vi "读写键段.vi"(7 "枚举":enum16{"write", "read", "读键", "读段"}(ring), 8 "值":string, 9 "key":string caption="键", 10 "段":string, 11 "配置文件":path=path "D:/Labviewprogram/多账户登录") -> (0 "读取值":string, 1 "键名":string[](array[string]) caption="获取键名", 2 "获取段名":string[](array[string]))   [LabVIEW 2018]
uses:
  <vilib>/Utility/config.llb/Write Key (String).vi
  <vilib>/Utility/config.llb/Read Key (String).vi
  <vilib>/Utility/config.llb/NI_LVConfig.lvlib
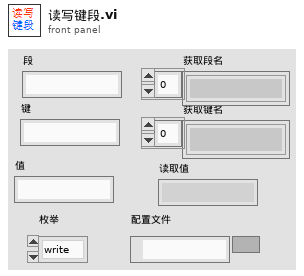
[diagram p1: front panel]
types:
  T1 = typedef "NI_LVConfig.lvlib/Config Data RefNum.ctl" = refnum<k1>
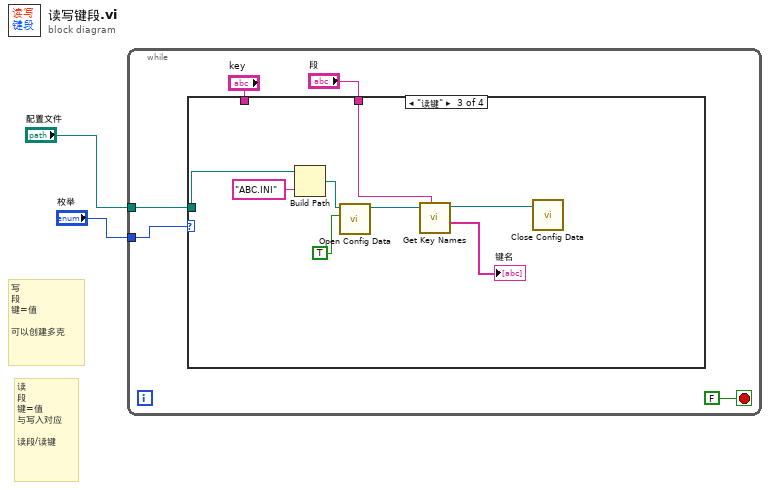
[diagram p0: block diagram]
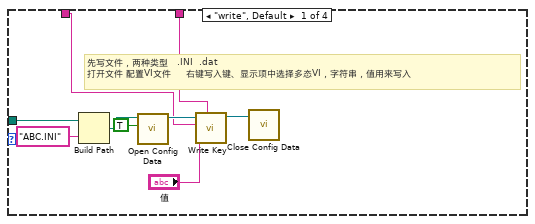
[diagram p2: hidden frame]
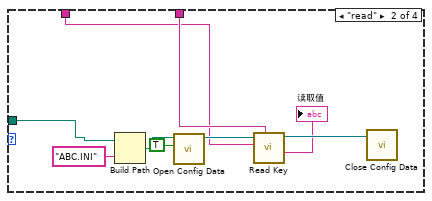
[diagram p3: hidden frame]
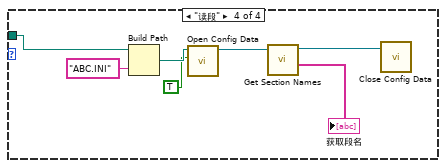
[diagram p4: hidden frame]
diagram:
  # "读\n段\n键=值\n与写入对应\n\n读段/读键"
  # "写\n段\n键=值\n\n可以创建多克"
  n1 = while {
    tunnel: "配置文件" -> [w5]
    tunnel: "枚举" -> [w6]
    stop <- FALSE stop-if-true
    n2 = case shown="\"读键\"" w6 {
      tunnel: w5 -> [w16 w20 w32 w34]
      tunnel: "段" -> [w10 w19 w27 _]
      tunnel: "key" -> [w9 w18 _ _]
      frame "write", Default {
        # "先写文件，两种类型   .INI  .dat\n打开文件 配置VI文件     右键写入键、显示项中选择多态VI，字符串，值用来写入"
        n3 = Build Path(base path=w16, name or relative path="ABC.INI" ("名称或相对路径")) -> (appended path=w14:path)
        n4 = call <vilib>:"Open Config Data.vi"("create file if necessary (T)"=TRUE, "configuration file path"=w14) -> ("refnum"=w13:T1)  [unwired: 7 in, 2 out]
        n5 = call-poly <vilib>:"Write Key.vi"("section"=w10, "value"="值", "key"=w9, "refnum"=w13) -> ("refnum out"=w12:T1)  [unwired: 5 in, 2 out]
        n6 = call <vilib>:"Close Config Data.vi"("refnum"=w12) -> ()  [unwired: 9 in, 2 out]
      }
      frame "read" {
        n7 = Build Path(base path=w20, name or relative path="ABC.INI" ("名称或相对路径")) -> (appended path=w25:path)
        n8 = call <vilib>:"Open Config Data.vi"("create file if necessary (T)"=TRUE, "configuration file path"=w25) -> ("refnum"=w24:T1)  [unwired: 7 in, 2 out]
        n9 = call-poly <vilib>:"Read Key.vi"("section"=w19, "key"=w18, "refnum"=w24) -> ("value"=→"读取值":string, "refnum out"=w23:T1)  [unwired: 5 in, 2 out]
        n10 = call <vilib>:"Close Config Data.vi"("refnum"=w23) -> ()  [unwired: 9 in, 2 out]
      }
      frame "读键" {
        n11 = Build Path(base path=w32, name or relative path="ABC.INI" ("名称或相对路径")) -> (appended path=w31:path)
        n12 = call <vilib>:"Open Config Data.vi"("create file if necessary (T)"=TRUE, "configuration file path"=w31) -> ("refnum"=w29:T1)  [unwired: 7 in, 2 out]
        n13 = call <vilib>:"Get Key Names.vi"("section"=w27, "refnum"=w29) -> ("key names"=→"键名":string[], "refnum out"=w28:T1)  [unwired: 6 in, 2 out]
        n14 = call <vilib>:"Close Config Data.vi"("refnum"=w28) -> ()  [unwired: 9 in, 2 out]
      }
      frame "读段" {
        n15 = Build Path(base path=w34, name or relative path="ABC.INI" ("名称或相对路径")) -> (appended path=w40:path)
        n16 = call <vilib>:"Open Config Data.vi"("create file if necessary (T)"=TRUE, "configuration file path"=w40) -> ("refnum"=w39:T1)  [unwired: 7 in, 2 out]
        n17 = call <vilib>:"Get Section Names.vi"("refnum"=w39) -> ("section names"=→"获取段名":string[], "refnum out"=w38:T1)  [unwired: 8 in, 1 out]
        n18 = call <vilib>:"Close Config Data.vi"("refnum"=w38) -> ()  [unwired: 9 in, 2 out]
      }
    }
  }
